vi "Set Fuel Valve Percent.vi"(8 "Error In":errorcluster, 10 "Percent":i32, 11 "ECU COM Port":refnum<visa-resource-name>) -> (0 "Error Out":errorcluster, 3 "ECU COM Port Out":refnum<visa-resource-name>)   [LabVIEW 2017]
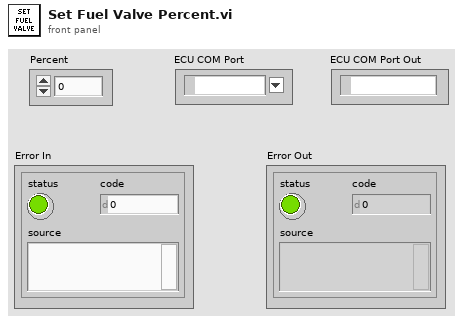
[diagram p1: front panel]
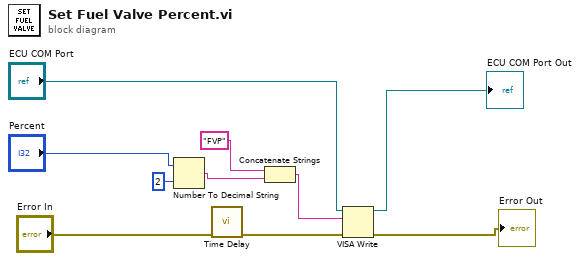
[diagram p0: block diagram]
diagram:
  n1 = Number To Decimal String(number="Percent", width (-)=i16 2) -> (decimal integer string=w9:string)
  n2 = call "Time Delay"("error in (no error)"="Error In") -> ("error out"=w2:errorcluster)  [unwired: 10 in]
  n3 = Concatenate Strings("FVP" ("write buffer"), w9) -> (w10:string)
  n4 = VISA Write(VISA resource name="ECU COM Port", write buffer=w10, error in (no error)=w2) -> (VISA resource name out=→"ECU COM Port Out":refnum<visa-resource-name>, error out=→"Error Out":errorcluster)  [unwired: 1 out]
